vi "NKT_STOP.vi"(8 "entrée d'erreur (pas d'erreur)":errorcluster) -> (0 "sortie d'erreur":errorcluster)   [LabVIEW 2026]
uses:
  <instrlib>/NKTP_API/NKTP_API.lvlib
  Controls/TypeDef_FGV.ctl
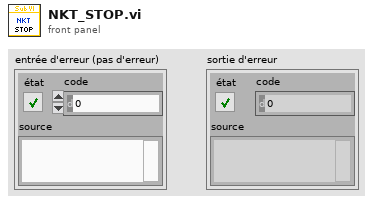
[diagram p1: front panel]
types:
  T1 = typedef "TypeDef_FGV.ctl" = enum16{"Initialize", "Write", "Read"}
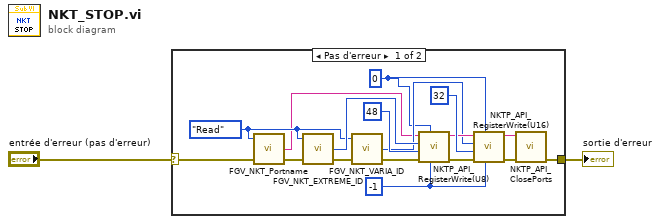
[diagram p0: block diagram]
diagram:
  n1 = case shown="Pas d'erreur" "entrée d'erreur (pas d'erreur)" {
    selector: "entrée d'erreur (pas d'erreur)" -> [w7 w20]
    tunnel: [w13 w20] -> w2
    frame No Error {
      w6 = TypeDef_FGV."Read" ("Action")
      w3 = i16 -1 ("index")
      w4 = u8 0 ("value")
      n2 = call "FGV_NKT_Portname.vi"("error in"=w7, "Action"=w6) -> ("error out"=w8:errorcluster, "Portname"=w5:string)  [unwired: 2 in]
      n3 = call "FGV_NKT_EXTREME_ID.vi"("error in"=w8, "Action"=w6) -> ("error out"=w12:errorcluster, "ID"=w11:i32)  [unwired: 2 in]
      n4 = call "FGV_NKT_VARIA_ID.vi"("error in"=w12, "Action"=w6) -> ("error out"=w9:errorcluster, "ID"=w10:i32)  [unwired: 2 in]
      n5 = call <instrlib>:"NKTP_API_RegisterWrite(U8).vi"("index"=w3, "value"=w4, "error in"=w9, "regId"=u8 48, "devId"=w11, "portname"=w5) -> ("error out"=w16:errorcluster, "portname out"=w15:string)  [unwired: 4 in]
      n6 = call <instrlib>:"NKTP_API_RegisterWrite(U16).vi"("index"=w3, "value"=w4, "error in"=w16, "regId"=u8 32, "devId"=w10, "portname"=w15) -> ("error out"=w19:errorcluster, "portname out"=w18:string)  [unwired: 4 in]
      n7 = call <instrlib>:"NKTP_API_ClosePorts.vi"("error in"=w19, "portnames"=w18) -> ("error out"=w13:errorcluster)  [unwired: 8 in, 1 out]
    }
    frame Error {
    }
  }
  "sortie d'erreur" <- w2
